vi "简易流程调试界面.vi"() -> ()   [LabVIEW 2016, in "斯坦道氨氮.lvlib"]
uses:
  <vilib>/Utility/miscctls.llb/LVPointTypeDef.ctl
  <vilib>/Plasmionique/MB Master/MB_Master/MB_Master.lvclass
panel:
  in  "调试控件":enum32{"填充流程", "清洗流程", "测试流程", "排空流程", "其他流程"}(tab)
  in  "填充简易流程":i32(listbox)
  in  "清洗简易流程":i32(listbox)
  in  "测试简易流程":i32(listbox)
  in  "排空简易流程":i32(listbox)
  in  "其他简易流程":i32(listbox)
  in  "停止":bool
  in  "单步测试":bool
  out "注射器温度":sgl
  out "消解温度":sgl
  out "ADC":sgl
  out "F3":sgl format="%#.6f"
  out "F2":sgl format="%#.6f"
  out "F1":sgl format="%#.6f"
  out "F0":sgl format="%#.6f"
  in  "启动":bool
  in  "参数下拉列表":u16(ring) items=["总磷"=1]
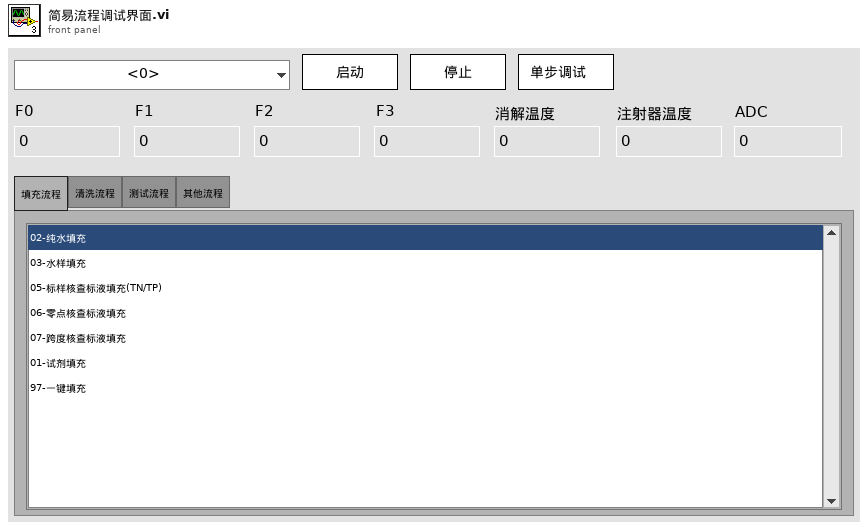
[diagram p1: front panel]
types:
  T1 = typedef "LVPointTypeDef.ctl" = cluster{"Horizontal":i16, "Vertical":i16}
  T2 = typedef "LVRectTypeDef.ctl" = cluster{"Left":i16, "Top":i16, "Right":i16, "Bottom":i16}
  T3 = typedef "LVStringsAndValuesArrayTypeDef_U16.ctl" = cluster{"String":string, "Value":u16}[]
  T4 = typedef "操作日志字段定义.ctl" = cluster{"时间":timestamp, "参数":string, "日志信息":string, "流程参数":string}
  T5 = enum16{"跨度核查", "水样测量", "零点核查", "标样核查", "加标回收", "快捷测试", "空白校准", "标样校准"}
  T6 = cluster{"系统时间":timestamp, "工作状态":u16, "测量模式":enum16{"待机", "连续模式", "周期模式", "定点模式", "受控模式", "手动模式"}, "告警代码":u16, "故障代码":u16, "日志代码":u16, "软件版本":u16, "F0":sgl, "F1":sgl, "F2":sgl, "F3":sgl, "T":sgl, "H":sgl, "id":u16, "flowid":u16, "量程":u16, "总磷控温温度1":sgl, "营养盐控温温度2":sgl, "ADC":sgl, "结果值":sgl, "运行时间":u16, "步骤详情":string, "步骤流程":string}
  T7 = typedef "SingleStepTestV3.lvlib/SingleStepTestV3.lvclass/仪器版本.ctl" = enum16{"V3.1版", "V4版", "V3版", "V4.2版"}
  T8 = enum32{"Bad", "Idle", "Run top level", "Running"}
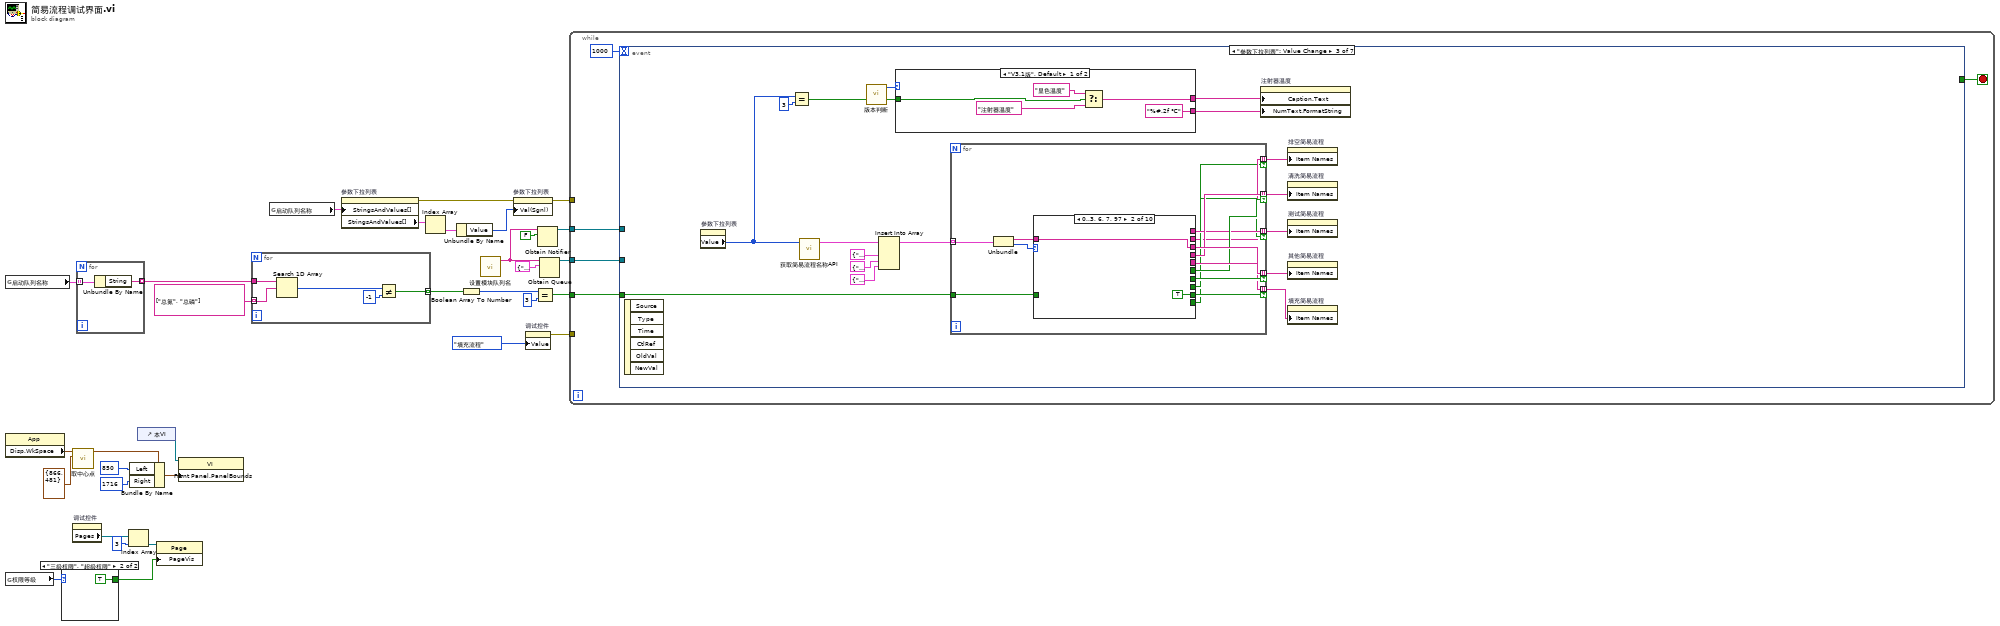
[diagram p0: block diagram]
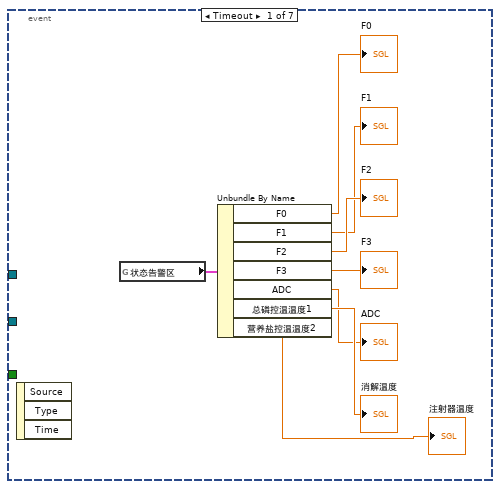
[diagram p3: hidden frame]
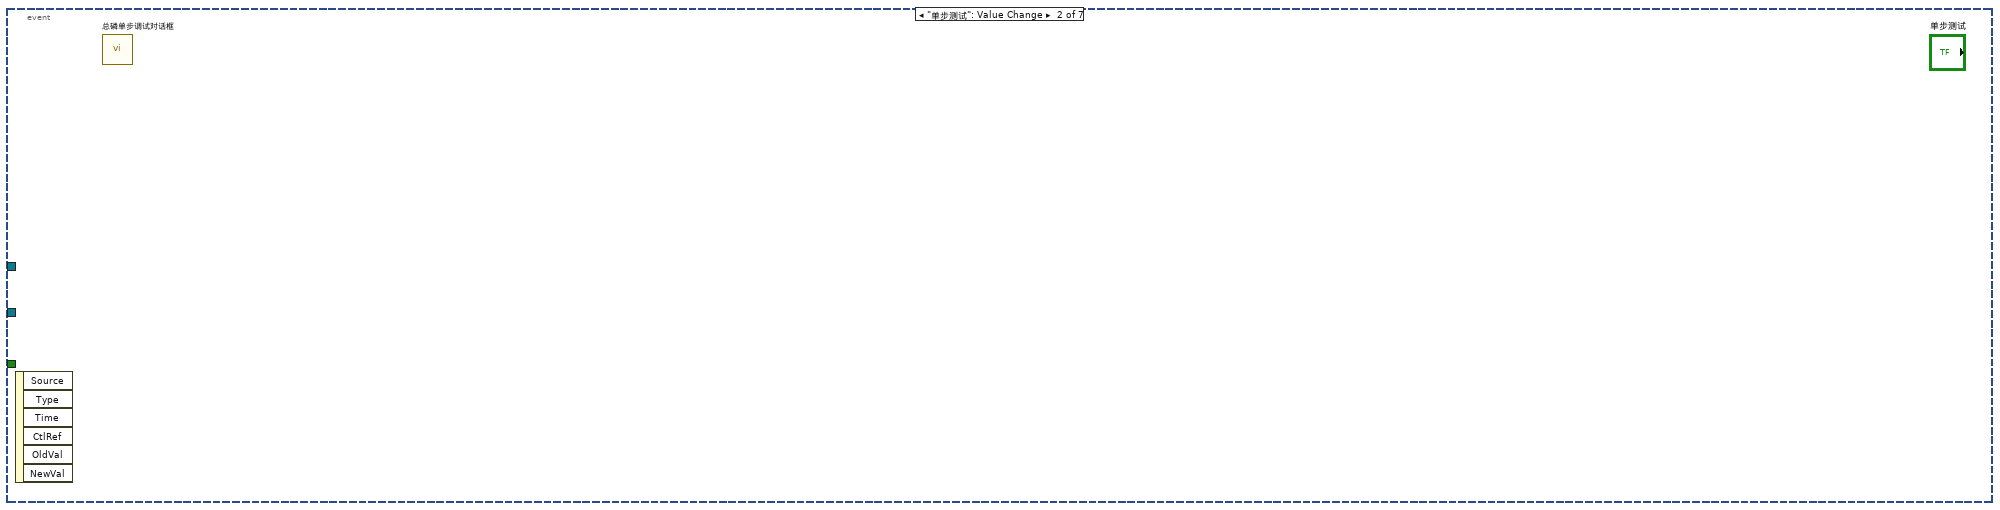
[diagram p4: hidden frame]
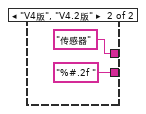
[diagram p5: hidden frame]
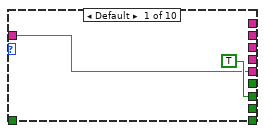
[diagram p6: hidden frame]
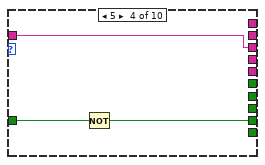
[diagram p8: hidden frame]
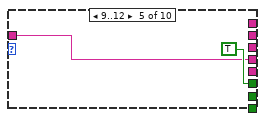
[diagram p9: hidden frame]
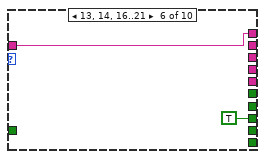
[diagram p10: hidden frame]
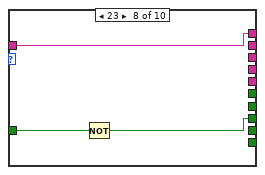
[diagram p12: hidden frame]
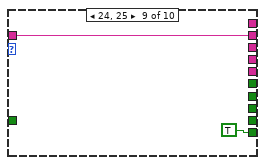
[diagram p13: hidden frame]
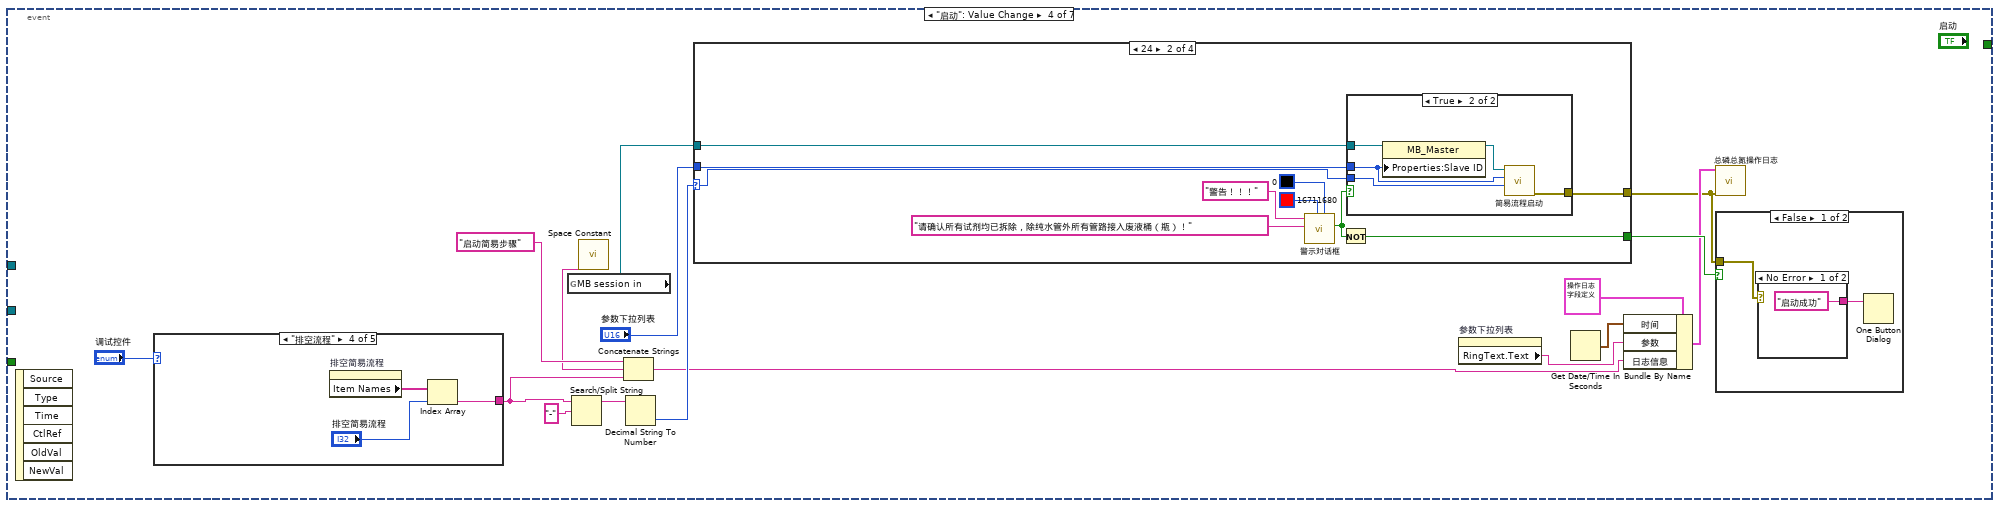
[diagram p15: hidden frame]
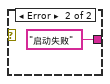
[diagram p16: hidden frame]
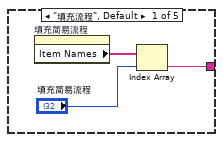
[diagram p18: hidden frame]
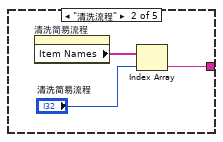
[diagram p19: hidden frame]
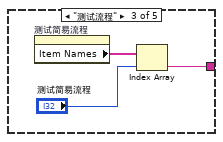
[diagram p20: hidden frame]
diagram:
  n1 = global read "model config var.vi" "启动队列名称"() -> (w3:cluster{"String":string, "Value":u16}[])
  n2 = property class="App"() -> ("Disp.WkSpace"=w13:T2)  [unwired: 2 in, 2 out]
  n3 = global read "VAR总磷总氮全局变量.vi" "权限等级"() -> (w19:enum16{"一级权限", "二级权限", "三级权限", "超级权限"})
  n4 = case shown="\"三级权限\", \"超级权限\"" w19 {
    tunnel: [_ TRUE ("选项卡可见")] -> w15
    frame "一级权限", Default {
    }
    frame "三级权限", "超级权限" {
    }
  }
  n5 = call "取中心点.vi"("前面板窗口:最小尺寸"=T1 {"Horizontal"=866, "Vertical"=481}, "显示:主工作区"=w13) -> ("前面板窗口:窗口边界"=w11:T2)  [unwired: 9 in]
  n6 = property on="调试控件" class="TabCtl (strict)"() -> ("Pages"=w18:refnum<vi>[])  [unwired: 2 in, 2 out]
  n7 = for {
    tunnel: w3 -> [w35] mode=indexing
    tunnel: [w34] -> w4 mode=indexing
    n8 = Unbundle By Name(w35) -> ("String"=w34:string)
  }
  n9 = Index Array(array=w18, index=3 ("索引")) -> (element=w16:refnum<vi>)
  n10 = Bundle By Name(cluster=w11, "Left"=i16 850, "Right"=i16 1716) -> (w10:T2)
  n11 = control-ref of="本VI"() -> (w14:refnum<vi>)
  n12 = property class="Page"(reference=w16, "PageVis"=w15) -> ()  [unwired: 1 in, 2 out]
  n13 = property class="VI"(reference=w14, "Front Panel.PanelBounds"=w10) -> ()  [unwired: 1 in, 2 out]
  n14 = for {
    tunnel: string[] ["总氮", "总磷"] -> [w39] mode=indexing
    tunnel: w4 -> [w40]
    tunnel: [w36] -> w5 mode=indexing
    n15 = Search 1D Array(1D array=w40, element=w39) -> (index of element=w38:i32)  [unwired: 1 in]
    n16 = Not Equal?(x=w38, y=-1) -> (x != y?=w36:bool)
  }
  n17 = global read "model config var.vi" "启动队列名称"() -> (w27:cluster{"String":string, "Value":u16}[])
  n18 = property on="参数下拉列表" class="Ring (strict)"("StringsAndValues[]"=w27) -> (error out=w28:errorcluster, "StringsAndValues[]"=w31:T3)  [unwired: 2 in, 1 out]
  n19 = Index Array(array=w31) -> (element=w30:cluster{"String":string, "Value":u16})  [unwired: 1 in]
  n20 = Unbundle By Name(w30) -> ("Value"=w29:u16)
  n21 = Boolean Array To Number(Boolean array=w5) -> (number=w6:u32)
  n22 = call "设置模块队列名.vi"() -> ("Msg"=w24:string)  [unwired: 5 in]
  n23 = property on="参数下拉列表" class="Ring (strict)"(error in=w28, "Val(Sgnl)"=w29) -> (error out=w32:errorcluster)  [unwired: 1 in, 1 out]
  n24 = property on="调试控件" class="TabCtl (strict)"("Value"=enum32{"填充流程", "清洗流程", "测试流程", "排空流程", "其他流程"}."填充流程" ("调试控件")) -> (error out=w20:errorcluster)  [unwired: 2 in, 1 out]
  n25 = Equal?(x=w6, y=u32 3) -> (x = y?=w1:bool)
  n26 = Obtain Notifier(name (unnamed)=w24, notification data type=FALSE) -> (notifier out=w23:refnum<notifier>)  [unwired: 2 in, 2 out]
  n27 = Obtain Queue(name (unnamed)=w24, element data type=cluster{"命令":string, "data":variant} {"命令"="", "data"=variant}) -> (queue out=w22:refnum<queue>)  [unwired: 3 in, 2 out]
  n28 = while {
    tunnel: w32 -> [_]
    tunnel: w23 -> [w43]
    tunnel: w22 -> [w42]
    tunnel: w20 -> [_]
    tunnel: w1 -> [w41]
    stop <- w45 stop-if-true
    n29 = event shown="[2] \"参数下拉列表\": Value Change" {
      selector: _ -> [_ _ _ _ _ _ _]
      dyn-events: _ -> [_ _ _ _ _ _ _]
      timeout: 1000 -> [_ _ _ _ _ _ _]
      tunnel: [_ _ _ _ _ _ TRUE] -> w45
      tunnel: w43 -> [_ _ _ _ _ w196 _]
      tunnel: w42 -> [_ _ _ _ _ w195 _]
      tunnel: w41 -> [_ _ w70 _ _ _ _]
      event Timeout {
        n30 = event-data() -> ()  [unwired: 1 in, 3 out]
        n31 = global read "VAR总磷总氮全局变量.vi" "状态告警区"() -> (w53:T6)
        n32 = Unbundle By Name(w53) -> ("F0"=→"F0":sgl, "F1"=→"F1":sgl, "F2"=→"F2":sgl, "F3"=→"F3":sgl, "ADC"=→"ADC":sgl, "总磷控温温度1"=→"消解温度":sgl, "营养盐控温温度2"=→"注射器温度":sgl)
      }
      event "单步测试": Value Change {
        n33 = event-data() -> ()  [unwired: 1 in, 6 out]
        n34 = call "总磷单步调试对话框.vi"() -> ()  [unwired: 12 in]
      }
      event "参数下拉列表": Value Change {
        n35 = event-data() -> ()  [unwired: 1 in, 6 out]
        n36 = property on="参数下拉列表" class="Ring (strict)"() -> ("Value"=w58:u16)  [unwired: 2 in, 2 out]
        n37 = Equal?(x=w58, y=u16 3) -> (x = y?=w56:bool)
        n38 = call "获取简易流程名称API.vi"("参数下拉列表"=w58) -> ("字符串与值[]"=w60:T3)  [unwired: 9 in, 1 out]
        n39 = call "版本判断.vi"() -> ("仪器版本"=w59:T7)  [unwired: 11 in]
        n40 = Insert Into Array(array=w60, new element #1=cluster{string, i32} {"97-一键填充", 97} ("新元素/子数组"), new element #2=cluster{string, i32} {"98-快捷测试（低量程）", 98} ("新元素/子数组"), new element #3=cluster{string, i32} {"99-快捷测试（高量程）", 99} ("新元素/子数组")) -> (w67:T3)  [unwired: 1 in]
        n41 = case shown="\"V3.1版\", Default" w59 {
          tunnel: [w71 "传感器" ("标题.文本")] -> w55
          tunnel: ["%#.2f ℃" ("数值文本.格式字符串") "%#.2f " ("数值文本.格式字符串")] -> w54
          tunnel: w56 -> [w74 _]
          frame "V3.1版", Default {
            n42 = Select(t="显色温度", s=w74, f="注射器温度" ("标题.文本")) -> (s? t:f=w71:string)
          }
          frame "V4版", "V4.2版" {
          }
        }
        n43 = for {
          tunnel: w67 -> [w90] mode=indexing
          tunnel: [w89] -> w65 mode=indexing if=w88
          tunnel: [w87] -> w64 mode=indexing if=w86
          tunnel: [w85] -> w63 mode=indexing if=w84
          tunnel: [w83] -> w62 mode=indexing if=w82
          tunnel: [w81] -> w61 mode=indexing if=w80
          tunnel: w70 -> [w79]
          n44 = Unbundle(w90) -> ("String"=w78:string, "Value"=w91:u16)
          n45 = case shown="0..3, 6, 7, 97" w91 {
            tunnel: [w92 _ _ _ _ _ _ _ _ _] -> w89
            tunnel: [TRUE _ _ _ _ _ _ _ _ _] -> w88
            tunnel: [_ w94 w96 w98 _ _ _ _ _ _] -> w87
            tunnel: [_ TRUE w97 w99 _ _ _ _ _ _] -> w86
            tunnel: [_ _ _ _ w101 _ _ _ _ _] -> w85
            tunnel: [_ _ _ _ TRUE _ _ _ _ _] -> w84
            tunnel: [_ _ _ _ _ w103 w105 w107 _ _] -> w83
            tunnel: [_ _ _ _ _ TRUE w106 w108 _ _] -> w82
            tunnel: [_ _ _ _ _ _ _ _ w110 w112] -> w81
            tunnel: [_ _ _ _ _ _ _ _ TRUE _] -> w80
            tunnel: w79 -> [_ _ w97 w100 _ _ w106 w109 _ _]
            tunnel: w78 -> [w92 w94 w96 w98 w101 w103 w105 w107 w110 w112]
            frame Default {
            }
            frame 0..3, 6, 7, 97 {
            }
            frame 4 {
            }
            frame 5 {
              n46 = Not(x=w100) -> (.not. x?=w99:bool)
            }
            frame 9..12 {
            }
            frame 13, 14, 16..21 {
            }
            frame 22 {
            }
            frame 23 {
              n47 = Not(x=w109) -> (.not. x?=w108:bool)
            }
            frame 24, 25 {
            }
            frame 8, 15 {
            }
          }
        }
        n48 = property on="注射器温度" class="DigNum (strict)"("Caption.Text"=w55, "NumText.FormatString"=w54) -> ()  [unwired: 2 in, 2 out]
        n49 = property on="排空简易流程" class="LstBox (strict)"("Item Names"=w61) -> ()  [unwired: 2 in, 2 out]
        n50 = property on="清洗简易流程" class="LstBox (strict)"("Item Names"=w63) -> ()  [unwired: 2 in, 2 out]
        n51 = property on="测试简易流程" class="LstBox (strict)"("Item Names"=w62) -> ()  [unwired: 2 in, 2 out]
        n52 = property on="其他简易流程" class="LstBox (strict)"("Item Names"=w65) -> ()  [unwired: 2 in, 2 out]
        n53 = property on="填充简易流程" class="LstBox (strict)"("Item Names"=w64) -> ()  [unwired: 2 in, 2 out]
      }
      event "启动": Value Change {
        n54 = event-data() -> ()  [unwired: 1 in, 6 out]
        n55 = case shown="\"排空流程\"" "调试控件" {
          tunnel: [w133 w136 w139 w142 w145] -> w114
          frame "填充流程", Default {
            n56 = property on="填充简易流程" class="LstBox (strict)"() -> ("Item Names"=w135:string[])  [unwired: 2 in, 2 out]
            n57 = Index Array(array=w135, index="填充简易流程") -> (element=w133:string)
          }
          frame "清洗流程" {
            n58 = property on="清洗简易流程" class="LstBox (strict)"() -> ("Item Names"=w138:string[])  [unwired: 2 in, 2 out]
            n59 = Index Array(array=w138, index="清洗简易流程") -> (element=w136:string)
          }
          frame "测试流程" {
            n60 = property on="测试简易流程" class="LstBox (strict)"() -> ("Item Names"=w141:string[])  [unwired: 2 in, 2 out]
            n61 = Index Array(array=w141, index="测试简易流程") -> (element=w139:string)
          }
          frame "排空流程" {
            n62 = property on="排空简易流程" class="LstBox (strict)"() -> ("Item Names"=w144:string[])  [unwired: 2 in, 2 out]
            n63 = Index Array(array=w144, index="排空简易流程") -> (element=w142:string)
          }
          frame "其他流程" {
            n64 = property on="其他简易流程" class="LstBox (strict)"() -> ("Item Names"=w147:string[])  [unwired: 2 in, 2 out]
            n65 = Index Array(array=w147, index="其他简易流程") -> (element=w145:string)
          }
        }
        n66 = global read "VAR总磷总氮全局变量.vi" "MB session in"() -> (w128:refnum<class "MB_Master.lvclass">)
        n67 = Search/Split String(string=w114, search string/char (-)="-" ("搜索字符串/字符(-)")) -> (substring before match=w124:string)  [unwired: 1 in, 2 out]
        n68 = call <vilib>:"Space Constant.vi"() -> ("String"=w113:string)
        n69 = Concatenate Strings("启动简易步骤" ("日志信息"), w113, w114) -> (w115:string)
        n70 = Decimal String To Number(string=w124) -> (number=w123:i32)  [unwired: 2 in, 1 out]
        n71 = case shown="24" w123 {
          selector: w123 -> [w150 w161 _ w182]
          tunnel: [w152 w162 _ w186] -> w116
          tunnel: w128 -> [w149 w160 _ w185]
          tunnel: "参数下拉列表" -> [w148 w159 w168 w184]
          tunnel: [_ w158 _ _] -> w122
          frame 0, Default {
            n72 = property class="MB_Master"(reference=w149, "Properties:Slave ID"=w148) -> (reference out=w151:refnum<class "MB_Master.lvclass">)  [unwired: 1 in, 1 out]
            n73 = call "简易流程启动.vi"("简易流程"=w150, "参数Id"=w148, "MB session in"=w151) -> ("error out"=w152:errorcluster)  [unwired: 7 in, 1 out]
          }
          frame 24 {
            n74 = call "警示对话框.vi"("副标题颜色"=u32 0, "主标题颜色"=u32 16711680, "副标题"="请确认所有试剂均已拆除，除纯水管外所有管路接入废液桶（瓶）！" ("消息"), "主标题"="警告！！！" ("消息")) -> ("check"=w153:bool)  [unwired: 7 in]
            n75 = Not(x=w153) -> (.not. x?=w158:bool)
            n76 = case shown="True" w153 {
              tunnel: [_ w167] -> w162
              tunnel: w161 -> [_ w165]
              tunnel: w160 -> [_ w164]
              tunnel: w159 -> [_ w163]
              frame False {
              }
              frame True {
                n77 = property class="MB_Master"(reference=w164, "Properties:Slave ID"=w163) -> (reference out=w166:refnum<class "MB_Master.lvclass">)  [unwired: 1 in, 1 out]
                n78 = call "简易流程启动.vi"("简易流程"=w165, "参数Id"=w163, "MB session in"=w166) -> ("error out"=w167:errorcluster)  [unwired: 7 in, 1 out]
              }
            }
          }
          frame 97 {
            n79 = vi-ref "一键清洗流程.vi"() -> (w169:refnum<vi>)
            n80 = property class="VI"(reference=w169) -> ("Name"=w170:string, "Exec.State"=w171:T8)  [unwired: 1 in, 2 out]
            n81 = case shown="\"Idle\"" w171 {
              tunnel: w170 -> [_ w180]
              tunnel: w168 -> [_ w173]
              frame "Bad", Default {
              }
              frame "Idle" {
                n82 = property on="填充简易流程" class="LstBox (strict)"() -> ("Item Names"=w172:string[])  [unwired: 2 in, 2 out]
                n83 = Open VI Reference(type specifier VI Refnum (for type only)=refnum<vi> refnum, vi path=w180, options=128 ("选项")) -> (vi reference=w177:refnum<vi>, error out=w175:errorcluster)  [unwired: 3 in]
                n84 = call-by-ref "开始异步调用"(reference=w177, error in=w175, "项名"=w172, "参数下拉列表"=w173) -> (reference out=w176:refnum<vi>, error out=w174:errorcluster)  [unwired: 10 in]
                n85 = Close Reference(reference=w176, error in (no error)=w174) -> ()  [unwired: 1 out]
              }
            }
          }
          frame 98, 99 {
            n86 = case shown="98, Default" w182 {
              tunnel: [enum16{"低量程", "高量程"}."低量程" ("量程下拉列表") enum16{"低量程", "高量程"}."高量程" ("量程下拉列表")] -> w181
              frame 98, Default {
              }
              frame 99 {
              }
            }
            n87 = call "非国标启动命令.vi"("参数下拉列表"=w184, "量程下拉列表"=w181, "测量模式"=T5."快捷测试", "MB session in"=w185) -> ("error out"=w186:errorcluster)  [unwired: 6 in, 1 out]
          }
        }
        n88 = property on="参数下拉列表" class="Ring (strict)"() -> ("RingText.Text"=w118:string)  [unwired: 2 in, 2 out]
        n89 = Get Date/Time In Seconds() -> (seconds since 1Jan1904=w119:timestamp)
        n90 = Bundle By Name(cluster=T4 {"时间"=timestamp(0 s since 1904-01-01), "参数"="", "日志信息"="", "流程参数"=""} ("data in"), "时间"=w119, "参数"=w118, "日志信息"=w115) -> (w120:T4)
        n91 = call "总磷总氮操作日志.vi"("错误输入（无错误）"=w116, "data in"=w120) -> ()  [unwired: 9 in, 1 out]
        n92 = case shown="False" w122 {
          tunnel: w116 -> [w130 _]
          frame False {
            n93 = case shown="No Error" w130 {
              tunnel: ["启动成功" "启动失败"] -> w129
              frame No Error {
              }
              frame Error {
              }
            }
            n94 = One Button Dialog(message=w129) -> ()  [unwired: 1 in, 1 out]
          }
          frame True {
          }
        }
      }
      event "排空简易流程": Mouse Down {
        n95 = event-data() -> ()  [unwired: 1 in, 6 out]
      }
      event "停止": Value Change {
        n96 = event-data() -> ()  [unwired: 1 in, 6 out]
        n97 = Send Notification(notification=TRUE ("通知"), notifier=w196) -> ()  [unwired: 1 in, 2 out]
        n98 = Enqueue Element(queue=w195, element=cluster{"命令":string, "data":variant} {"命令"="启动", "data"=variant(cluster{"站号":u16, "控制命令输出":u16[]} {"站号"=1, "控制命令输出"=[2816]})} ("元素")) -> (queue out=w198:refnum<queue>)  [unwired: 2 in, 2 out]
        n99 = property on="参数下拉列表" class="Ring (strict)"() -> ("RingText.Text"=w189:string)  [unwired: 2 in, 2 out]
        n100 = Get Date/Time In Seconds() -> (seconds since 1Jan1904=w192:timestamp)
        n101 = Enqueue Element(queue=w198, element=cluster{"命令":string, "data":variant} {"命令"="启动", "data"=variant(cluster{"站号":u16, "控制命令输出":u16[]} {"站号"=2, "控制命令输出"=[2816]})} ("元素")) -> (error out=w190:errorcluster)  [unwired: 2 in, 2 out]
        n102 = Bundle By Name(cluster=T4 {"时间"=timestamp(0 s since 1904-01-01), "参数"="", "日志信息"="", "流程参数"=""} ("data in"), "时间"=w192, "参数"=w189, "日志信息"="手动停止") -> (w193:T4)
        n103 = call "总磷总氮操作日志.vi"("错误输入（无错误）"=w190, "data in"=w193) -> ()  [unwired: 9 in, 1 out]
      }
      event Panel Close {
        n104 = event-data() -> ()  [unwired: 1 in, 3 out]
      }
    }
  }
